vi "Save Dicom.vi"(6 "Enum":enum16{"Save Image", "Load Image"}(ring)=enum."Load Image", 8 "Error in":errorcluster, 10 "Data Cluster":T1, 11 "Input Image":T2) -> (0 "Error out":errorcluster, 3 "Output Image":T2)   [LabVIEW 2021]
uses:
  <vilib>/vision/Image Controls.llb/IMAQ Image.ctl
  <userlib>/_MGI/Error Reporter/MGI Error Reporter Base/MGI Error Reporter Base.lvclass
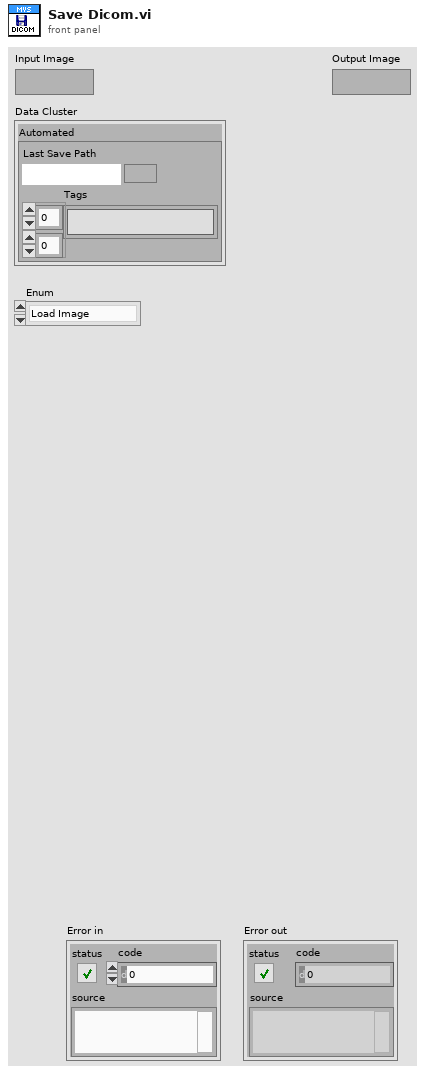
[diagram p1: front panel]
types:
  T1 = cluster{"Automated":cluster{"Last Save Path":path, "Tags":string[][]}}
  T2 = typedef "IMAQ Image.ctl" = refnum<image>
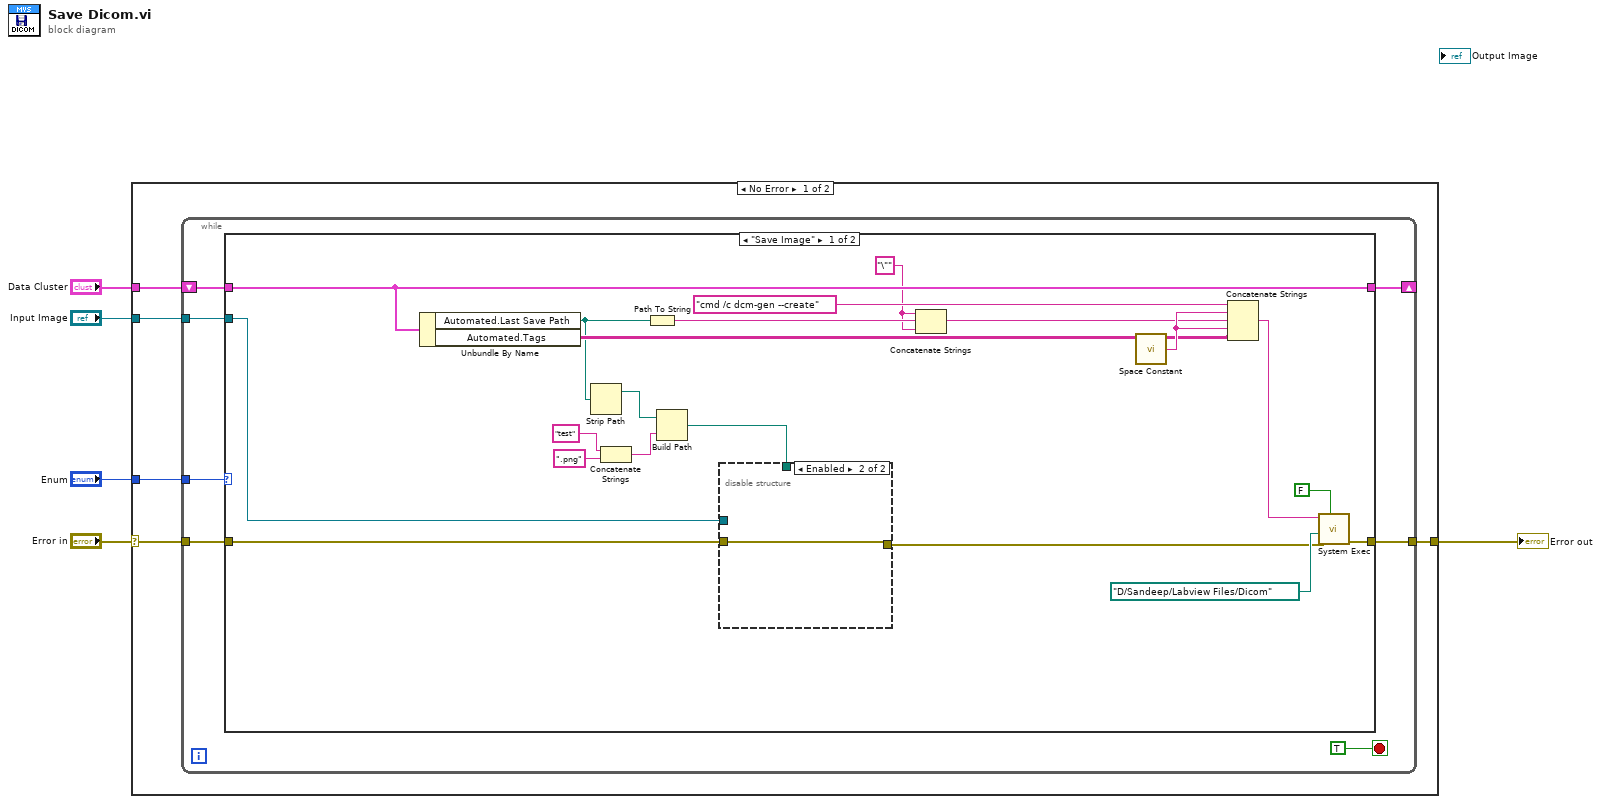
[diagram p0: block diagram]
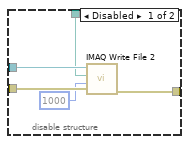
[diagram p2: hidden frame]
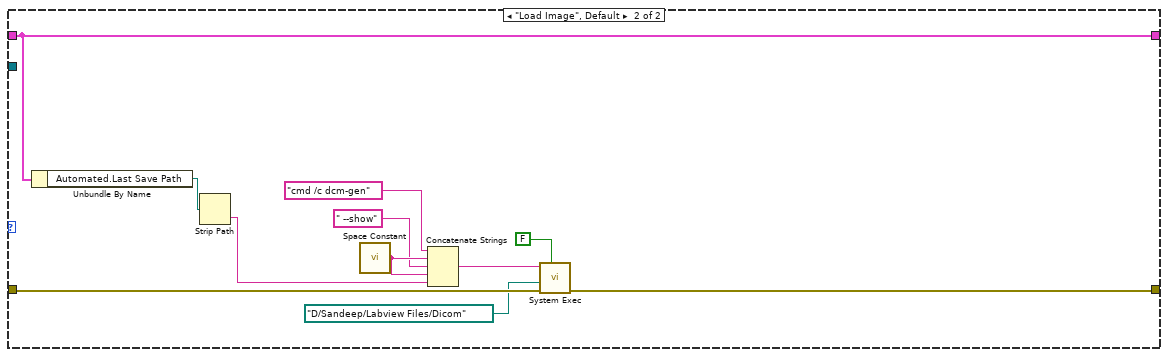
[diagram p3: hidden frame]
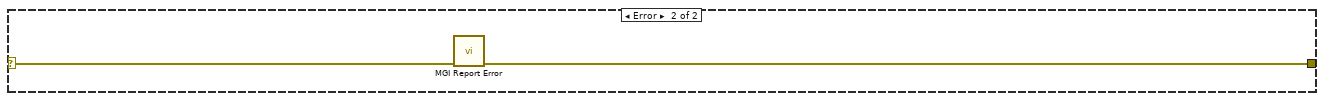
[diagram p4: hidden frame]
diagram:
  n1 = case shown="No Error" "Error in" {
    selector: "Error in" -> [w9 w56]
    tunnel: "Data Cluster" -> [w10 _]
    tunnel: [w8 w55] -> w4
    tunnel: "Enum" -> [w6 _]
    tunnel: "Input Image" -> [w7 _]
    frame No Error {
      n2 = while {
        shift-right: [w16] -> _
        shift-left: w10 -> [w17]
        tunnel: w9 -> [w15]
        tunnel: [w14] -> w8
        tunnel: w7 -> [w13]
        tunnel: w6 -> [w11]
        stop <- TRUE stop-if-true
        n3 = case shown="\"Save Image\"" w11 {
          tunnel: w17 -> [w35 w51]
          tunnel: [w35 w51] -> w16
          tunnel: [w37 w54] -> w14
          tunnel: w15 -> [w29 w49]
          tunnel: w13 -> [w30 _]
          frame "Save Image" {
            w26 = "\""
            n4 = Unbundle By Name(w35) -> ("Automated.Last Save Path"=w23:path, "Automated.Tags"=w24:string[][])
            n5 = Strip Path(path=w23) -> (stripped path=w22:path)  [unwired: 1 out]
            n6 = Concatenate Strings("test" ("string"), ".png") -> (w21:string)
            n7 = Path To String(path=w23) -> (string=w28:string)
            n8 = Build Path(base path=w22, name or relative path=w21) -> (appended path=w18:path)
            n9 = disable-structure shown="Enabled" {
              disable-tunnel: w30 -> [w42 _]
              disable-tunnel: w29 -> [w41 w43]
              disable-tunnel: [w39 w43] -> w25
              disable-tunnel: w18 -> [w38 _]
              frame Disabled {
                n10 = call-poly "IMAQ Write File 2"("error in (no error)"=w41, "Image Quality"=u32 1000, "File Path"=w38, "Image"=w42) -> ("error out"=w39:errorcluster)  [unwired: 6 in, 1 out]
              }
              frame Enabled {
              }
            }
            n11 = Concatenate Strings(w26, w28, w26) -> (w27:string)
            n12 = call <vilib>:"Space Constant.vi"() -> ("String"=w32:string)
            n13 = Concatenate Strings("cmd /c dcm-gen --create" ("string"), w32, w27, w32, w24) -> (w36:string)
            n14 = call <vilib>:"System Exec.vi"("wait until completion? (T)"=FALSE, "error in (no error)"=w25, "working directory"=path "D:/Sandeep/Labview Files/Dicom", "command line"=w36) -> ("error out"=w37:errorcluster)  [unwired: 4 in, 3 out]
          }
          frame "Load Image", Default {
            n15 = Unbundle By Name(w51) -> ("Automated.Last Save Path"=w50:path)
            n16 = Strip Path(path=w50) -> (name=w47:string)  [unwired: 1 out]
            n17 = call <vilib>:"Space Constant.vi"() -> ("String"=w46:string)
            n18 = Concatenate Strings("cmd /c dcm-gen" ("string"), w46, " --show" ("string"), w46, w47) -> (w52:string)
            n19 = call <vilib>:"System Exec.vi"("wait until completion? (T)"=FALSE, "error in (no error)"=w49, "working directory"=path "D:/Sandeep/Labview Files/Dicom", "command line"=w52) -> ("error out"=w54:errorcluster)  [unwired: 4 in, 3 out]
          }
        }
      }
    }
    frame Error {
      n20 = call <userlib>:"MGI Report Error.vi"("error in"=w56) -> ("no error"=w55:errorcluster)  [unwired: 10 in]
    }
  }
  "Error out" <- w4
